vi "Freq to Period.vi"(11 "PWMFrequency":i32) -> (3 "Period (dt)":i64)   [LabVIEW 2019, in "HVC6.lvlib" / "HVC6.lvclass"]
uses:
  HVC6 Class/HVC6.lvclass
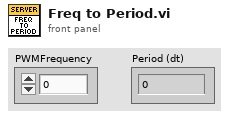
[diagram p1: front panel]
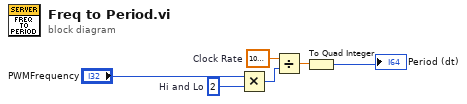
[diagram p0: block diagram]
diagram:
  w1 = i64 2  # Hi and Lo
  w3 = 1000000.0  # Clock Rate
  n1 = Multiply(x="PWMFrequency", y=w1) -> (x*y=w2:i64)
  n2 = Divide(x=w3, y=w2) -> (x/y=w5:dbl)
  n3 = To Quad Integer(1:w5) -> (0:→"Period (dt)":i64)
